vi "FirstSteps.vi"() -> ()   [LabVIEW 2012]
uses:
  <instrlib>/TCxxxx/TCxxxx.lvlib
panel:
  out "Return Count 2":u32
  out "Return Count":u32
  out "Read Buffer 11":string
  out "Read Buffer 10":string
  in  "Write Buffer 10":string="\u0015"
  out "Read Buffer 9":string
  out "Read Buffer 8":string
  out "Read Buffer 7":string
  in  "Write Buffer 9":string="0"
  in  "Write Buffer 8":string="0"
  in  "Write Buffer 7":string="1"
  out "Read Buffer 6":string
  in  "Write Buffer 6":string="_"
  out "Read Buffer 5":string
  out "Read Buffer 4":string
  in  "Write Buffer 5":string="0"
  in  "Write Buffer 4":string="_"
  out "Read Buffer 3":string
  in  "Write Buffer 3":string="w"
  out "Read Buffer 2":string
  in  "Write Buffer 2":string="_"
  in  "Write Buffer":string="**A"
  out "error out":errorcluster
  in  "VISA resource name":refnum<visa-resource-name>
  out "Read Buffer":string
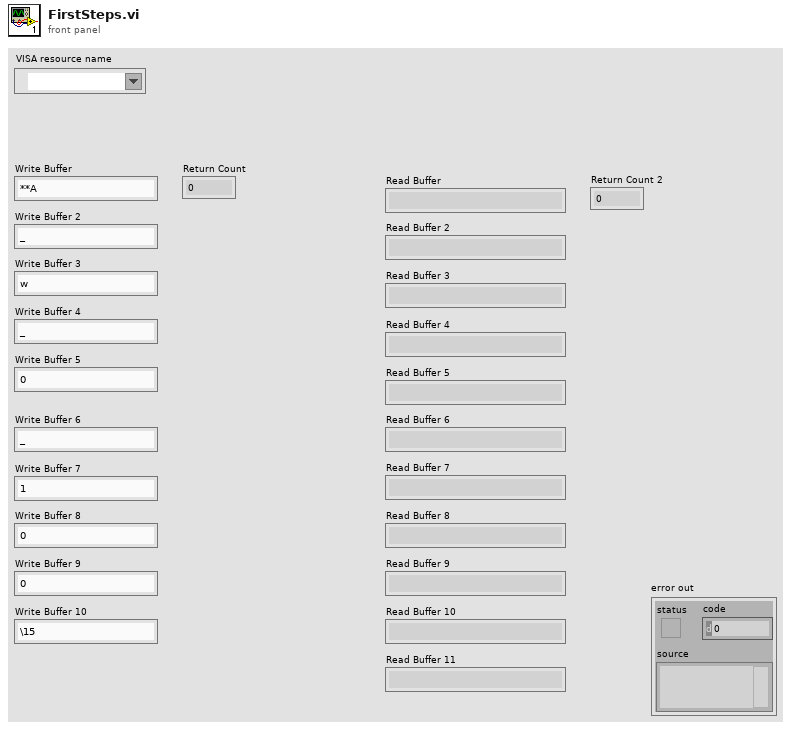
[diagram p1: front panel]
types:
  T1 = cluster{"Baud Rate":u32, "Parity":u16, "Data Bits":u16, "Stop Bits":u16, "Flow Control":u16}
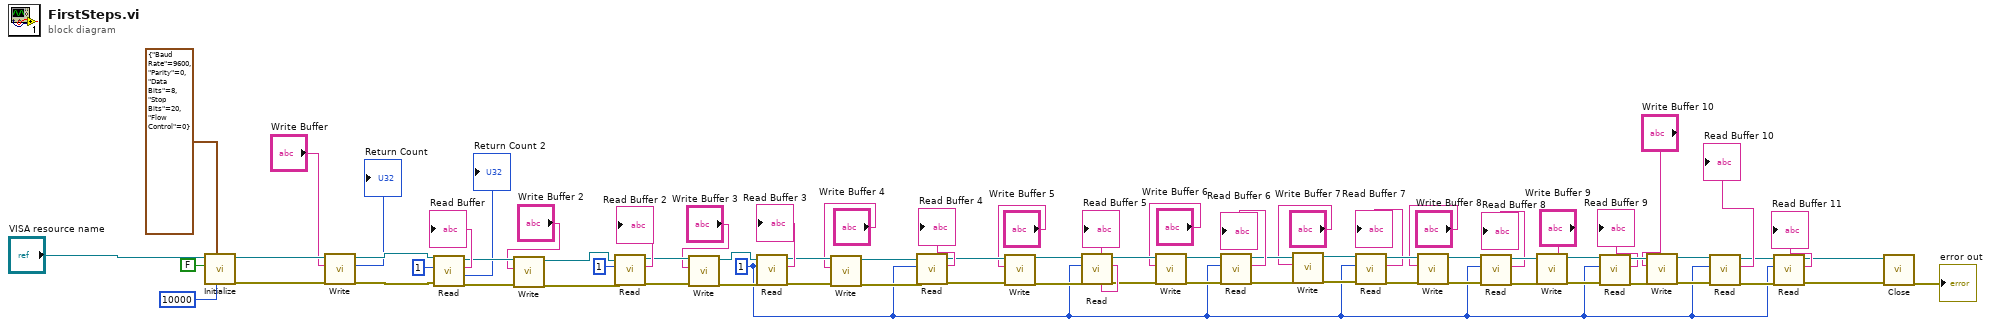
[diagram p0: block diagram]
diagram:
  w3 = u32 1 ("Byte Count")
  n1 = call <instrlib>:"Initialize.vi"("Timeout [ms]"=u32 10000, "Serial Configuration"=T1 {"Baud Rate"=9600, "Parity"=0, "Data Bits"=8, "Stop Bits"=20, "Flow Control"=0}, "ID Query (True)"=FALSE, "VISA resource name"="VISA resource name") -> ("error out"=w60:errorcluster, "VISA resource name out"=w63:refnum<visa-resource-name>)  [unwired: 6 in]
  n2 = call <instrlib>:"Write.vi"("error in (no error)"=w60, "Write Buffer"="Write Buffer", "VISA resource name"=w63) -> ("error out"=w61:errorcluster, "Return Count"=→"Return Count":u32, "VISA resource name out"=w62:refnum<visa-resource-name>)  [unwired: 6 in]
  n3 = call <instrlib>:"Read.vi"("error in (no error)"=w61, "Byte Count"=u32 1, "VISA resource name"=w62) -> ("error out"=w57:errorcluster, "Return Count"=→"Return Count 2":u32, "Read Buffer"=→"Read Buffer":string, "VISA resource name out"=w58:refnum<visa-resource-name>)  [unwired: 5 in]
  n4 = call <instrlib>:"Write.vi"("error in (no error)"=w57, "Write Buffer"="Write Buffer 2", "VISA resource name"=w58) -> ("error out"=w54:errorcluster, "VISA resource name out"=w55:refnum<visa-resource-name>)  [unwired: 6 in, 1 out]
  n5 = call <instrlib>:"Read.vi"("error in (no error)"=w54, "Byte Count"=u32 1, "VISA resource name"=w55) -> ("error out"=w52:errorcluster, "Read Buffer"=→"Read Buffer 2":string, "VISA resource name out"=w53:refnum<visa-resource-name>)  [unwired: 5 in, 1 out]
  n6 = call <instrlib>:"Write.vi"("error in (no error)"=w52, "Write Buffer"="Write Buffer 3", "VISA resource name"=w53) -> ("error out"=w50:errorcluster, "VISA resource name out"=w51:refnum<visa-resource-name>)  [unwired: 6 in, 1 out]
  n7 = call <instrlib>:"Read.vi"("error in (no error)"=w50, "Byte Count"=w3, "VISA resource name"=w51) -> ("error out"=w48:errorcluster, "Read Buffer"=→"Read Buffer 3":string, "VISA resource name out"=w45:refnum<visa-resource-name>)  [unwired: 5 in, 1 out]
  n8 = call <instrlib>:"Write.vi"("error in (no error)"=w48, "Write Buffer"="Write Buffer 4", "VISA resource name"=w45) -> ("error out"=w47:errorcluster, "VISA resource name out"=w46:refnum<visa-resource-name>)  [unwired: 6 in, 1 out]
  n9 = call <instrlib>:"Read.vi"("error in (no error)"=w47, "Byte Count"=w3, "VISA resource name"=w46) -> ("error out"=w43:errorcluster, "Read Buffer"=→"Read Buffer 4":string, "VISA resource name out"=w40:refnum<visa-resource-name>)  [unwired: 5 in, 1 out]
  n10 = call <instrlib>:"Write.vi"("error in (no error)"=w43, "Write Buffer"="Write Buffer 5", "VISA resource name"=w40) -> ("error out"=w42:errorcluster, "VISA resource name out"=w41:refnum<visa-resource-name>)  [unwired: 6 in, 1 out]
  n11 = call <instrlib>:"Read.vi"("error in (no error)"=w42, "Byte Count"=w3, "VISA resource name"=w41) -> ("error out"=w37:errorcluster, "Read Buffer"=→"Read Buffer 5":string, "VISA resource name out"=w38:refnum<visa-resource-name>)  [unwired: 5 in, 1 out]
  n12 = call <instrlib>:"Write.vi"("error in (no error)"=w37, "Write Buffer"="Write Buffer 6", "VISA resource name"=w38) -> ("error out"=w35:errorcluster, "VISA resource name out"=w36:refnum<visa-resource-name>)  [unwired: 6 in, 1 out]
  n13 = call <instrlib>:"Read.vi"("error in (no error)"=w35, "Byte Count"=w3, "VISA resource name"=w36) -> ("error out"=w28:errorcluster, "Read Buffer"=→"Read Buffer 6":string, "VISA resource name out"=w32:refnum<visa-resource-name>)  [unwired: 5 in, 1 out]
  n14 = call <instrlib>:"Write.vi"("error in (no error)"=w28, "Write Buffer"="Write Buffer 7", "VISA resource name"=w32) -> ("error out"=w27:errorcluster, "VISA resource name out"=w31:refnum<visa-resource-name>)  [unwired: 6 in, 1 out]
  n15 = call <instrlib>:"Read.vi"("error in (no error)"=w27, "Byte Count"=w3, "VISA resource name"=w31) -> ("error out"=w26:errorcluster, "Read Buffer"=→"Read Buffer 7":string, "VISA resource name out"=w30:refnum<visa-resource-name>)  [unwired: 5 in, 1 out]
  n16 = call <instrlib>:"Write.vi"("error in (no error)"=w26, "Write Buffer"="Write Buffer 8", "VISA resource name"=w30) -> ("error out"=w25:errorcluster, "VISA resource name out"=w29:refnum<visa-resource-name>)  [unwired: 6 in, 1 out]
  n17 = call <instrlib>:"Read.vi"("error in (no error)"=w25, "Byte Count"=w3, "VISA resource name"=w29) -> ("error out"=w23:errorcluster, "Read Buffer"=→"Read Buffer 8":string, "VISA resource name out"=w22:refnum<visa-resource-name>)  [unwired: 5 in, 1 out]
  n18 = call <instrlib>:"Write.vi"("error in (no error)"=w23, "Write Buffer"="Write Buffer 9", "VISA resource name"=w22) -> ("error out"=w24:errorcluster, "VISA resource name out"=w21:refnum<visa-resource-name>)  [unwired: 6 in, 1 out]
  n19 = call <instrlib>:"Read.vi"("error in (no error)"=w24, "Byte Count"=w3, "VISA resource name"=w21) -> ("error out"=w17:errorcluster, "Read Buffer"=→"Read Buffer 9":string, "VISA resource name out"=w18:refnum<visa-resource-name>)  [unwired: 5 in, 1 out]
  n20 = call <instrlib>:"Write.vi"("error in (no error)"=w17, "Write Buffer"="Write Buffer 10", "VISA resource name"=w18) -> ("error out"=w19:errorcluster, "VISA resource name out"=w20:refnum<visa-resource-name>)  [unwired: 6 in, 1 out]
  n21 = call <instrlib>:"Read.vi"("error in (no error)"=w19, "Byte Count"=w3, "VISA resource name"=w20) -> ("error out"=w7:errorcluster, "Read Buffer"=→"Read Buffer 10":string, "VISA resource name out"=w8:refnum<visa-resource-name>)  [unwired: 5 in, 1 out]
  n22 = call <instrlib>:"Read.vi"("error in (no error)"=w7, "Byte Count"=w3, "VISA resource name"=w8) -> ("error out"=w1:errorcluster, "Read Buffer"=→"Read Buffer 11":string, "VISA resource name out"=w2:refnum<visa-resource-name>)  [unwired: 5 in, 1 out]
  n23 = call <instrlib>:"Close.vi"("error in (no error)"=w1, "VISA resource name"=w2) -> ("error out"=→"error out":errorcluster)  [unwired: 9 in]
